vi "tsdiag_set_s3_servertime.vi"(8 "error in (no error)":errorcluster, 9 "ATimeMs":i32, 10 "ADiagModuleIndex":i32, 11 "路径输入":path) -> (0 "error out":errorcluster, 2 "return":i32, 3 "路径输出":path)   [LabVIEW 2014]
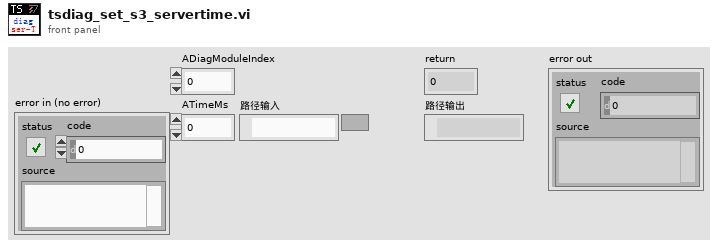
[diagram p1: front panel]
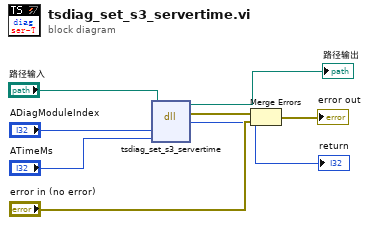
[diagram p0: block diagram]
diagram:
  n1 = dll-call lib="D:/Program Files (x86)/TOSUN/TSMaster/bin/TSMaster.dll" fn="tsdiag_set_s3_servertime"(path in="路径输入", "ADiagModuleIndex"="ADiagModuleIndex", "ATimeMs"="ATimeMs") -> (path out=→"路径输出":path, error out=w8:errorcluster, "ACode"=→"return":i32)  [unwired: 4 in]
  n2 = Merge Errors(w8, "error in (no error)") -> (→"error out":errorcluster)
